vi "Rate Limited Motor Speed.vi"() -> ()   [LabVIEW 2012]
doc: "<B>Rate Limited Motor Speed</B> sets a maximum rate of change for motor speed. It also displays the current speed and adjusts the desired speed in order to demonstrate the limited rate of change."
uses:
  <vilib>/Rock Robotics/SystemInterfaces/Typedef/FPGA_TypedefDigitalModule.ctl
  <vilib>/Rock Robotics/SystemInterfaces/DIO/FPGA_DIOPWMChannel.ctl
  <vilib>/Rock Robotics/WPI/MotorControl/WPI_MotorControlOpen Victor.vi
panel:
  in  "Maximum \nSpeed Change":dbl(knob) scale=0.0..2.0
  out "Current Speed":dbl(knob) scale=-1.0..1.0
  out "Victor LED":bool
  in  "Desired Speed (-1 to 1)":dbl(knob) min=-1.0 max=1.0 step=0.1 scale=-1.0..1.0 scale format="%#.3f"
  in  "PWM Channel":T1
  in  "DIO Module":T2
  in  "stop":bool
  # "Wiring Diagram for Digital Sidecar connected to an NI 9403"
  # "Set these inputs before running."
  # "This can be set while running."
  # "Digital Sidecar"
  # "Power\nTerminals"
  # "Motor\nTerminals"
  # "PWM cable"
  # "This shows wiring for a Victor speed controller.  The wiring is similar for a Luminary Micro Jaguar speed controller.  For a Jaguar, you must also select the appropriate instance of the Motor Open VI on the diagram."
  # "V-"
  # "M-"
  # "V+"
  # "M+"
  # "B"
  # "Innovation First"
  # "VICTOR 884"
  # "B"
  # "C"
  # "PWR"
  # "SIG"
  # "(-)"
  # "+V"
  # "10"
  # "9"
  # "8"
  # "7"
  # "6"
  # "5"
  # "4"
  # "3"
  # "2"
  # "1"
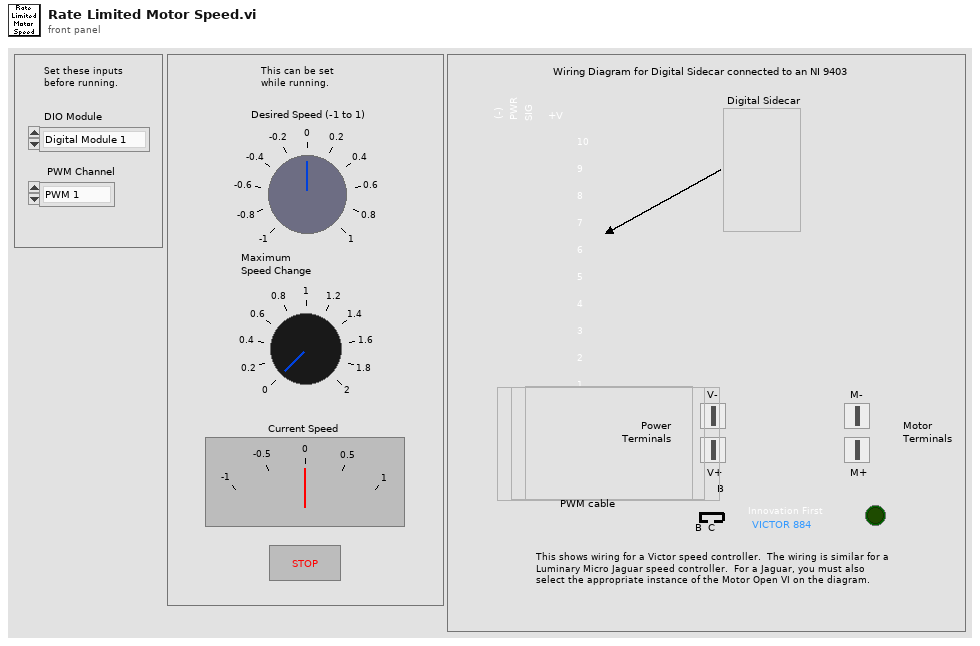
[diagram p1: front panel]
types:
  T1 = typedef "FPGA_DIOPWMChannel.ctl" = enum8{"PWM 1", "PWM 2", "PWM 3", "PWM 4", "PWM 5", "PWM 6", "PWM 7", "PWM 8", "PWM 9", "PWM 10", "Invalid"}
  T2 = typedef "FPGA_TypedefDigitalModule.ctl" = enum16{"Digital Module 1", "Digital Module 2"}
  T3 = typedef "WPI_MotorControlDeviceRef.ctl" = cluster{"DeviceStatus":errorcluster, "Type":enum16{"PWM", "CAN"}, "PWM":cluster{"Digital Module":T2, "PWM Channel":T1, "DeadBand":T4}, "CAN":cluster{"Device Number":u8, "Control Mode":T5, "Semaphore":T6, "Max Vout":dbl}, "Invert":bool, "TransformRef":T7, "InvTransformRef":T7}
  T4 = typedef "WPI_PWMDeadband.ctl" = cluster{"Name":string, "maxPositivePwm":i32, "minPositivePwm":i32, "centerPwm":i32, "maxNegativePwm":i32, "minNegativePwm":i32, "angularRange":u16}
  T5 = typedef "WPI_CANJaguar_ControlMode.ctl" = enum8{"Percent VBus", "Current", "Speed", "Position", "Voltage"}
  T6 = typedef "Semaphore RefNum" = refnum<k1>
  T7 = typedef "WPI_PWMTransform_ConPane.ctl" = refnum<vi>
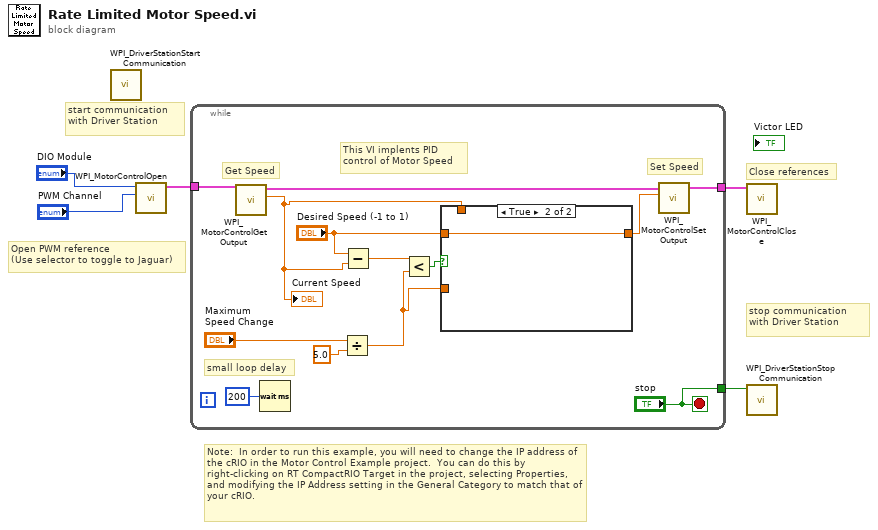
[diagram p0: block diagram]
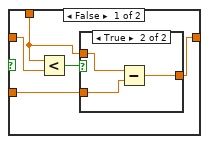
[diagram p2: hidden frame]
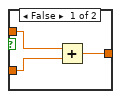
[diagram p3: hidden frame]
diagram:
  # "stop communication with Driver Station"
  # "start communication with Driver Station"
  # "Note:  In order to run this example, you will need to change the IP address of the cRIO in the Motor Control Example project.  You can do this by right-clicking on RT CompactRIO Target in the project, selecting Properties, and modifying the IP Address setting in the General Category to match that of your cRIO."
  # "Close references"
  # "Open PWM reference\n(Use selector to toggle to Jaguar)"
  n1 = call <vilib>:"WPI_DriverStationStart Communication.vi"() -> ()  [unwired: 1 in, 11 out]
  n2 = call-poly <vilib>:"WPI_MotorControlOpen.vi"("PWM Channel"="PWM Channel", "Digital Module (Module 1)"="DIO Module") -> ("MotorControlDeviceRef"=w3:T3)  [unwired: 5 in, 4 out]
  n3 = while {
    tunnel: w3 -> [w15]
    tunnel: [w18] -> w4
    tunnel: ["stop"] -> w5
    stop <- "stop" stop-if-true
    # "This VI implents PID\ncontrol of Motor Speed"
    # "Get Speed"
    # "small loop delay"
    # "Set Speed"
    n4 = call <vilib>:"WPI_MotorControlGetOutput.vi"("MotorControlDevRef"=w15) -> ("Output"=w7:dbl, "MotorControlDevRef"=w14:T3)  [unwired: 8 in, 1 out]
    "Current Speed" <- w7
    n5 = Wait (ms)(milliseconds to wait=u32 200) -> ()  [unwired: 1 out]
    n6 = Divide(x="Maximum \nSpeed Change", y=5.0) -> (x/y=w6:dbl)
    n7 = Subtract(x="Desired Speed (-1 to 1)", y=w7) -> (x-y=w13:dbl)
    n8 = Less?(x=w13, y=w6) -> (x < y?=w10:bool)
    n9 = case shown="True" w10 {
      tunnel: "Desired Speed (-1 to 1)" -> [w23 w30]
      tunnel: [w19 w30] -> w8
      tunnel: w7 -> [w21 _]
      tunnel: w6 -> [w20 _]
      frame False {
        n10 = Less?(x=w21, y=w23) -> (x < y?=w22:bool)
        n11 = case shown="True" w22 {
          tunnel: w21 -> [w25 w29]
          tunnel: w20 -> [w24 w28]
          tunnel: [w26 w27] -> w19
          frame False {
            n12 = Add(x=w25, y=w24) -> (x+y=w26:dbl)
          }
          frame True {
            n13 = Subtract(x=w29, y=w28) -> (x-y=w27:dbl)
          }
        }
      }
      frame True {
      }
    }
    n14 = call <vilib>:"WPI_MotorControlSetOutput.vi"("Output"=w8, "MotorControlDevRef"=w14) -> ("MotorControlDevRef"=w18:T3)  [unwired: 3 in, 6 out]
  }
  n15 = call <vilib>:"WPI_MotorControlClose.vi"("MotorControlDevRef"=w4) -> ()  [unwired: 1 in, 10 out]
  n16 = call <vilib>:"WPI_DriverStationStop Communication.vi"("StopCommunication"=w5) -> ()  [unwired: 1 in, 10 out]
